vi "dfd_Move Coef Quantizer Forward.vi"(1 "quantizers":T1[](array[typedef]) {"source" items=["Coefficients a/k"=0, "Coefficients b/v"=7, "Input"=1, "Output"=2, "Multiplicand"=3, "Product"=4, "Sum"=5, "Delay"=6]}) -> (0 "sorted quantizers":T1[](array[typedef]) {"source" items=["Coefficients a/k"=0, "Coefficients b/v"=7, "Input"=1, "Output"=2, "Multiplicand"=3, "Product"=4, "Sum"=5, "Delay"=6]})   [LabVIEW 2017, in "NI_DigFilter_FXP.lvlib"]
uses:
  <vilib>/addons/Digital Filter Design/NI_DigFilter_FXP.lvlib
  <vilib>/addons/Digital Filter Design/_Objects.llb/DFD Quantization Settings.ctl
  <vilib>/addons/Digital Filter Design/_Objects.llb/DFD Quantization Sources.ctl
  <vilib>/addons/Digital Filter Design/NI_DigFilterLicensed.lvlib
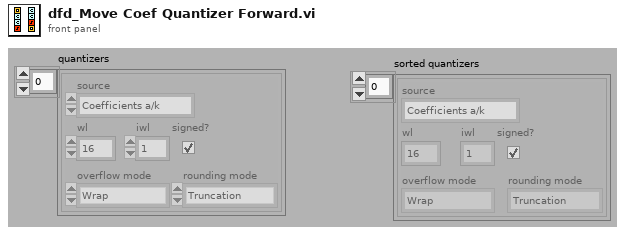
[diagram p1: front panel]
types:
  T1 = typedef "NI_DigFilterLicensed.lvlib/DFD Quantization Settings.ctl" = cluster{"source":T2, "wl":i16, "iwl":i16, "overflow mode":enum16{"Saturation", "Wrap"}, "rounding mode":enum16{"Nearest", "Truncation"}, "signed?":bool}
  T2 = typedef "NI_DigFilterLicensed.lvlib/DFD Quantization Sources.ctl" = u16
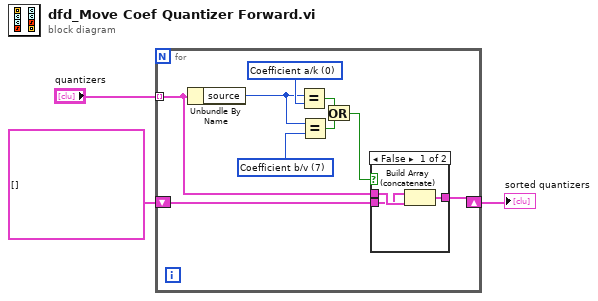
[diagram p0: block diagram]
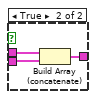
[diagram p2: hidden frame]
diagram:
  n1 = for {
    shift-right: [w4] -> w1
    shift-left: T1[] [] ("quantizers") -> [w6]
    tunnel: "quantizers" -> [w5] mode=indexing
    w10 = T2 7 items=["Coefficient a/k"=0, "Coefficient b/v"=7, "Input"=1, "Output"=2, "Multiplicand"=3, "Product"=4, "Sum"=5, "Delay"=6] ("y")
    w12 = T2 0 items=["Coefficient a/k"=0, "Coefficient b/v"=7, "Input"=1, "Output"=2, "Multiplicand"=3, "Product"=4, "Sum"=5, "Delay"=6] ("y")
    n2 = Unbundle By Name(w5) -> ("source"=w11:T2)
    n3 = Equal?(x=w11, y=w12) -> (x = y?=w9:bool)
    n4 = Equal?(x=w11, y=w10) -> (x = y?=w8:bool)
    n5 = Or(x=w9, y=w8) -> (x .or. y?=w7:bool)
    n6 = case shown="False" w7 {
      tunnel: w6 -> [w14 w18]
      tunnel: w5 -> [w15 w17]
      tunnel: [w13 w16] -> w4
      frame False {
        n7 = Build Array (concatenate)(w14, w15) -> (w13:T1[])
      }
      frame True {
        n8 = Build Array (concatenate)(w17, w18) -> (w16:T1[])
      }
    }
  }
  "sorted quantizers" <- w1
